vi "75_Vision_RC Servo_DC_Moto_3.vi"() -> ()   [LabVIEW 2018]
uses:
  <userlib>/KNR OS 4.0 LabVIEW Toolkit/Type Definition/Resource.ctl
  <userlib>/KNR OS 4.0 LabVIEW Toolkit/Type Definition/RC Servo Port.ctl
  <userlib>/KNR OS 4.0 LabVIEW Toolkit/Type Definition/DC Motor Port.ctl
panel:
  out "area":dbl
  out "RC Pulse Width (uS)":u16[](array[numeric])
  out "Image Out":T1(plugin-control)
  in  "stop":bool
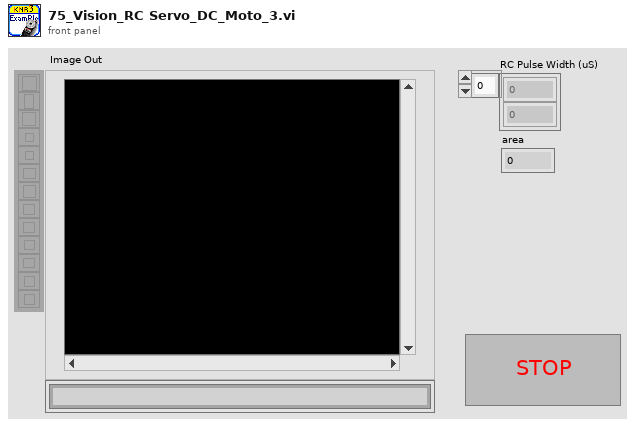
[diagram p1: front panel]
types:
  T1 = typedef "IMAQ Image.ctl" = refnum<image>
  T2 = typedef "DC Motor Port.ctl" = u16
  T3 = typedef "RC Servo Port.ctl" = u16
  T4 = typedef "Resource.ctl" = enum16{"KNRm_DDRC", "KNRm_DDDD", "KNRm_DDDR", "KNRm_DDDC", "KNR", "KNRm_neww"}
  T5 = typedef "KNR3 Reference.ctl" = cluster{"FPGA Session":refnum<class "FPGA Interface Base.lvclass">, "Resource":T4}
  T6 = cluster{"Left":dbl, "Top":dbl, "Right":dbl, "Bottom":dbl}
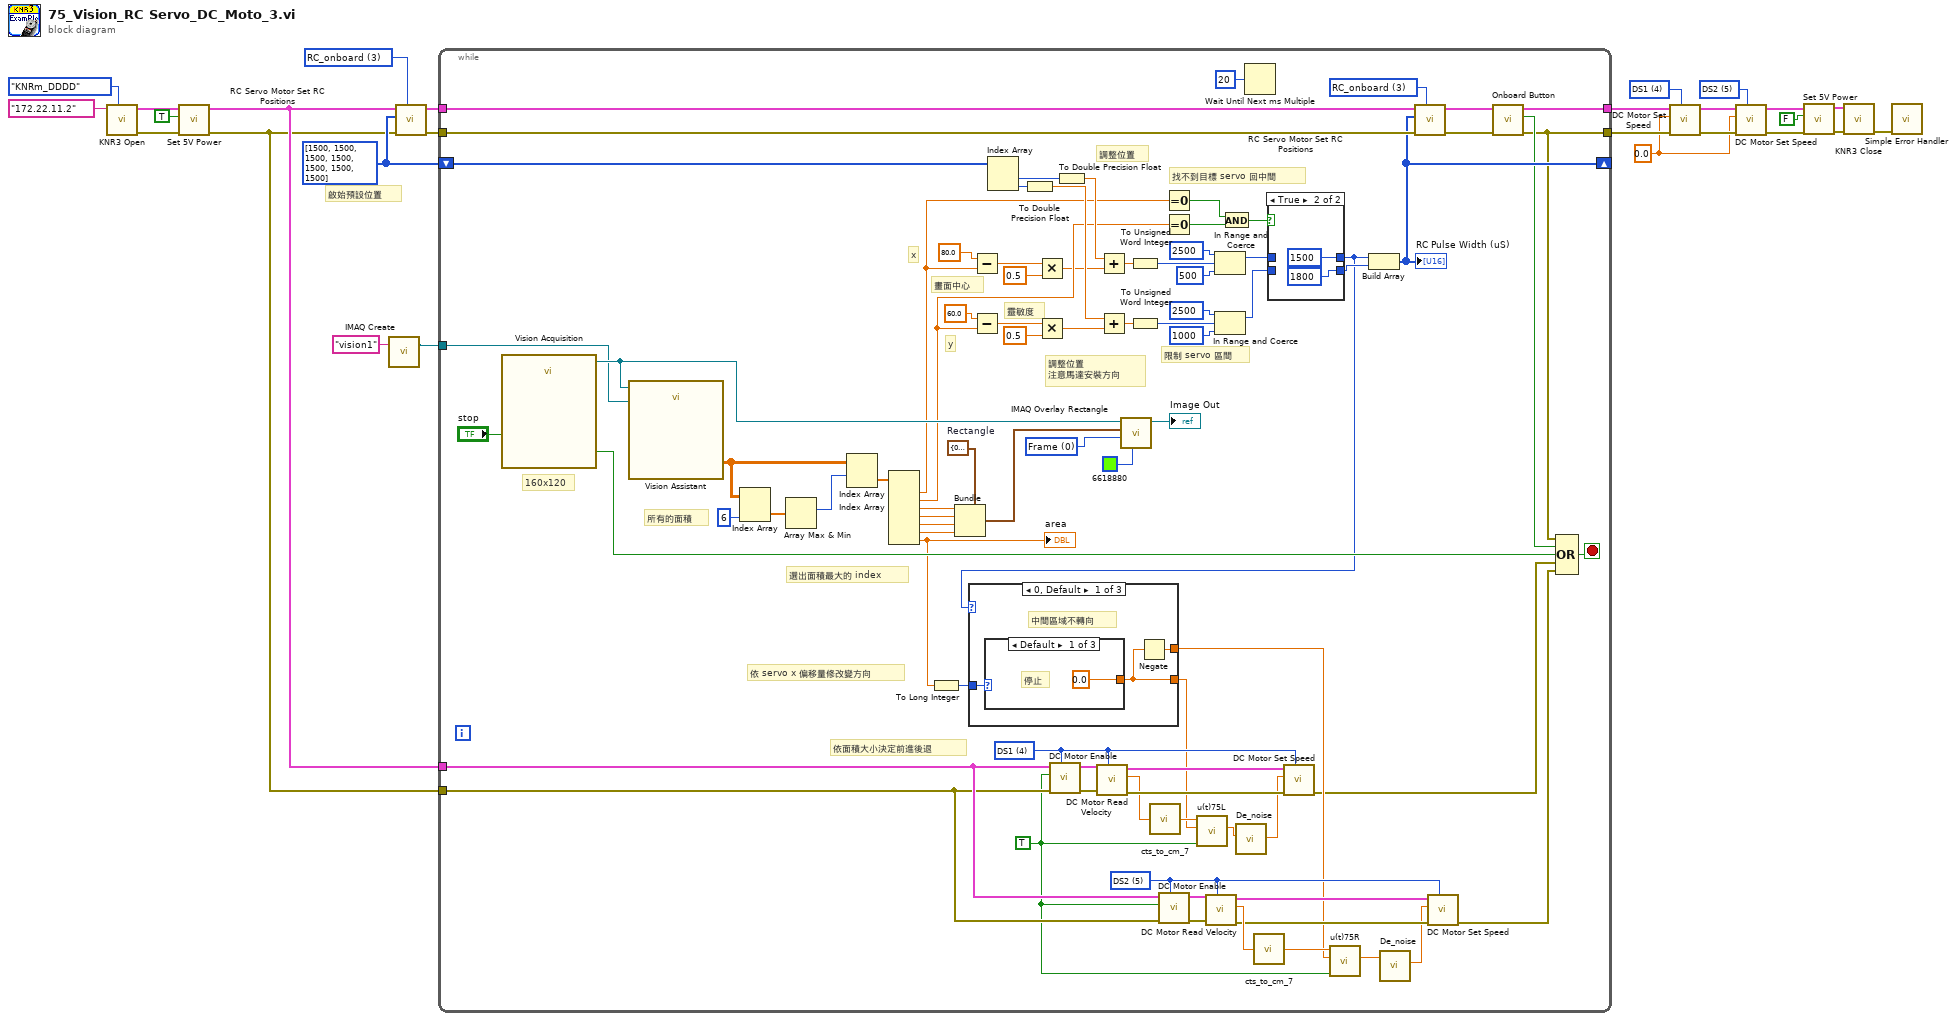
[diagram p0: block diagram]
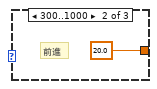
[diagram p2: hidden frame]
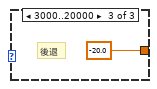
[diagram p3: hidden frame]
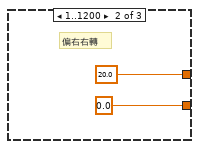
[diagram p4: hidden frame]
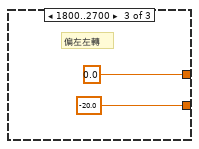
[diagram p5: hidden frame]
diagram:
  w1 = T2 5 items=["DS1"=4, "DS2"=5, "DS3"=6, "DS4"=7] ("Port (DS1)")
  w2 = T2 4 items=["DS1"=4, "DS2"=5, "DS3"=6, "DS4"=7] ("Port (DS1)")
  w3 = 0.0 ("Speed (+-100%)")
  w13 = u16[] [1500, 1500, 1500, 1500, 1500, 1500, 1500] ("RC Pulse Width (1500 uS)")
  w16 = T3 3 items=["RC_onboard"=3, "RC_box"=9] ("Port (RC_onboard)")
  # "啟始預設位置"
  n1 = call <userlib>:"KNR3 Open.vi"("Resource"=Resource."KNRm_DDDD", "IP"="172.22.11.2") -> ("error out"=w22:errorcluster, "KNR out"=w23:T5)  [unwired: 8 in]
  n2 = call <userlib>:"Set 5V Power.vi"("error in (no error)"=w22, "5V Power(T)"=TRUE ("5V Power"), "KNR in"=w23) -> ("error out"=w11:errorcluster, "KNR out"=w12:T5)  [unwired: 7 in]
  n3 = call "IMAQ Create"("Image Name"="vision1") -> ("New Image"=w14:T1)  [unwired: 4 in, 1 out]
  n4 = call <userlib>:"RC Servo Motor Set RC Positions.vi"("Port (RC_onboard)"=w16, "RC Pulse Width (1500 uS)"=w13, "KNR in"=w12) -> ("KNR out"=w17:T5)  [unwired: 7 in, 1 out]
  n5 = while {
    tunnel: w17 -> [w108]
    tunnel: [w35] -> w10
    tunnel: w11 -> [w106]
    tunnel: [w33] -> w9
    tunnel: w14 -> [w88]
    shift-right: [w72] -> _
    shift-left: w13 -> [w75]
    tunnel: w12 -> [w40]
    tunnel: w11 -> [w39]
    stop <- w105 stop-if-true
    w38 = u32 0 items=["Frame", "Fill", "Highlight"] ("Drawing Mode (Frame)")
    w42 = T2 5 items=["DS1"=4, "DS2"=5, "DS3"=6, "DS4"=7] ("Port 2")
    w36 = TRUE ("Enable Motor(F)")
    w55 = T2 4 items=["DS1"=4, "DS2"=5, "DS3"=6, "DS4"=7] ("Port 2")
    w101 = T6 {"Left"=0.0, "Top"=0.0, "Right"=0.0, "Bottom"=0.0}  # Rectangle
    w103 = T3 3 items=["RC_onboard"=3, "RC_box"=9] ("RC Motor")
    # "依 servo x 偏移量修改變方向"
    # "依面積大小決定前進後退"
    # "調整位置\n注意馬達安裝方向"
    # "調整位置"
    # "靈敏度"
    # "所有的面積"
    # "畫面中心"
    # "限制 servo 區間"
    # "找不到目標 servo 回中間"
    # "y"
    # "x"
    # "160x120"
    # "選出面積最大的 index"
    n6 = call "Vision Acquisition"("Stop (F)"="stop") -> ("Image Out"=w93:T1, "Stopped"=w86:bool)  [unwired: 24 in, 1 out]
    n7 = call "Vision Assistant"("Image In"=w93, "Image Dst"=w88) -> ("Particle Measurements (Pixels) (Particle Analysis 1)"=w92:dbl[][])  [unwired: 22 in, 3 out]
    n8 = Index Array "Index Array"(array=w92, index (col)=6 ("disabled index (col)")) -> (element=w91:dbl[])  [unwired: 1 in]
    n9 = Array Max & Min(array=w91) -> (max index (indices)=w90:i32)  [unwired: 3 out]
    n10 = Index Array "Index Array"(array=w92, index (row)=w90) -> (element=w102:dbl[])  [unwired: 1 in]
    n11 = Index Array "Index Array"(array=w102) -> (element #1=w65:dbl, element #2=w64:dbl, element #3=w100:dbl, element #4=w99:dbl, element #5=w98:dbl, element #6=w97:dbl, element #7=w49:dbl)  [unwired: 7 in]
    "area" <- w49
    n12 = To Long Integer(number=w49) -> (32bit integer=w27:i32)
    n13 = Bundle "Bundle"(cluster=w101, "Left"=w100, "Top"=w99, "Right"=w98, "Bottom"=w97) -> (w96:T6)
    n14 = Subtract(x=80.0 ("y"), y=w65) -> (x-y=w82:dbl)
    n15 = Subtract(x=60.0 ("y"), y=w64) -> (x-y=w83:dbl)
    n16 = Index Array "Index Array"(array=w75) -> (element #1=w74:u16, element #2=w73:u16)  [unwired: 2 in]
    n17 = To Double Precision Float(number=w73) -> (double precision float=w66:dbl)
    n18 = Multiply(x=w82, y=0.5) -> (x*y=w63:dbl)
    n19 = Multiply(x=w83, y=0.5) -> (x*y=w62:dbl)
    n20 = call <userlib>:"DC Motor Enable.vi"("Port (DS1)"=w55, "error in (no error)"=w39, "Enable Motor(F)"=w36, "KNR in"=w40) -> ("error out"=w51:errorcluster, "KNR out"=w50:T5)  [unwired: 6 in]
    n21 = To Double Precision Float(number=w74) -> (double precision float=w67:dbl)
    n22 = call <userlib>:"DC Motor Read Velocity.vi"("Port (DS1)"=w55, "error in (no error)"=w51, "KNR in"=w50) -> ("error out"=w54:errorcluster, "Velocity (cts/sec)"=w52:dbl, "KNR out"=w53:T5)  [unwired: 6 in]
    n23 = Add(x=w67, y=w63) -> (x+y=w84:dbl)
    n24 = Add(x=w66, y=w62) -> (x+y=w85:dbl)
    n25 = call "IMAQ Overlay Rectangle"("Color"=u32 6618880, "Drawing Mode (Frame)"=w38, "Rectangle"=w96, "Image"=w93) -> ("Image Out"=→"Image Out":T1)  [unwired: 6 in, 1 out]
    n26 = To Unsigned Word Integer(number=w84) -> (unsigned 16bit integer=w69:u16)
    n27 = To Unsigned Word Integer(number=w85) -> (unsigned 16bit integer=w68:u16)
    n28 = call "cts_to_cm_7.vi"("cts"=w52) -> ("cm"=w37:dbl)
    n29 = call <userlib>:"DC Motor Enable.vi"("Port (DS1)"=w42, "error in (no error)"=w39, "Enable Motor(F)"=w36, "KNR in"=w40) -> ("error out"=w46:errorcluster, "KNR out"=w47:T5)  [unwired: 6 in]
    n30 = Equal To 0?(x=w65) -> (x = 0?=w59:bool)
    n31 = Equal To 0?(x=w64) -> (x = 0?=w60:bool)
    n32 = call <userlib>:"DC Motor Read Velocity.vi"("Port (DS1)"=w42, "error in (no error)"=w46, "KNR in"=w47) -> ("error out"=w43:errorcluster, "Velocity (cts/sec)"=w45:dbl, "KNR out"=w44:T5)  [unwired: 6 in]
    n33 = In Range and Coerce(upper limit=u16 2500, x=w69, lower limit=u16 500) -> (coerced(x)=w58:u16)  [unwired: 1 out]
    n34 = In Range and Coerce(upper limit=u16 2500, x=w68, lower limit=u16 1000) -> (coerced(x)=w57:u16)  [unwired: 1 out]
    n35 = And(x=w59, y=w60) -> (x .and. y?=w61:bool)
    n36 = Wait Until Next ms Multiple(millisecond multiple=u32 20) -> ()  [unwired: 1 out]
    n37 = call "cts_to_cm_7.vi"("cts"=w45) -> ("cm"=w48:dbl)
    n38 = case shown="True" w61 {
      tunnel: w58 -> [w120 _]
      tunnel: w57 -> [w119 _]
      tunnel: [w120 u16 1500] -> w28
      tunnel: [w119 u16 1800] -> w56
      frame False {
      }
      frame True {
      }
    }
    n39 = case shown="0, Default" w28 {
      tunnel: [w110 0.0 -20.0] -> w26
      tunnel: [w111 20.0 0.0] -> w25
      tunnel: w27 -> [w109 _ _]
      frame 0, Default {
        # "中間區域不轉向"
        n40 = case shown="Default" w109 {
          tunnel: [0.0 20.0 -20.0] -> w110
          frame Default {
            # "停止"
          }
          frame 300..1000 {
            # "前進"
          }
          frame 3000..20000 {
            # "後退"
          }
        }
        n41 = Negate(x=w110) -> (-x=w111:dbl)
      }
      frame 1..1200 {
        # "偏右右轉"
      }
      frame 1800..2700 {
        # "偏左左轉"
      }
    }
    n42 = call "u(t)75L.vi"("Velocity"=w37, "Desire Velosity"=w26, "enable"=w36) -> ("u(t)"=w31:dbl)  [unwired: 7 in]
    n43 = call "De_noise.vi"("u(t)"=w31) -> ("u(t)2"=w32:dbl)  [unwired: 6 in]
    n44 = call <userlib>:"DC Motor Set Speed.vi"("Port (DS1)"=w55, "error in (no error)"=w54, "Speed (+-100%)"=w32, "KNR in"=w53) -> ("error out"=w24:errorcluster)  [unwired: 6 in, 1 out]
    n45 = call "u(t)75R.vi"("Velocity"=w48, "Desire Velosity"=w25, "enable"=w36) -> ("u(t)"=w30:dbl)  [unwired: 7 in]
    n46 = Build Array "Build Array"(w28, w56) -> (w72:u16[])
    "RC Pulse Width (uS)" <- w72
    n47 = call "De_noise.vi"("u(t)"=w30) -> ("u(t)2"=w29:dbl)  [unwired: 6 in]
    n48 = call <userlib>:"RC Servo Motor Set RC Positions.vi"("Port (RC_onboard)"=w103, "error in (no error)"=w106, "RC Pulse Width (1500 uS)"=w72, "KNR in"=w108) -> ("error out"=w33:errorcluster, "KNR out"=w107:T5)  [unwired: 6 in]
    n49 = call <userlib>:"DC Motor Set Speed.vi"("Port (DS1)"=w42, "error in (no error)"=w43, "Speed (+-100%)"=w29, "KNR in"=w44) -> ("error out"=w41:errorcluster)  [unwired: 6 in, 1 out]
    n50 = call <userlib>:"Onboard Button.vi"("KNR in"=w107) -> ("value"=w34:bool, "KNR out"=w35:T5)  [unwired: 8 in, 1 out]
    n51 = Compound Arithmetic op=OR(w33, w34, w86, w24, w41) -> (w105:bool)
  }
  n52 = call <userlib>:"DC Motor Set Speed.vi"("Port (DS1)"=w2, "Speed (+-100%)"=w3, "KNR in"=w10) -> ("KNR out"=w5:T5)  [unwired: 7 in, 1 out]
  n53 = call <userlib>:"DC Motor Set Speed.vi"("Port (DS1)"=w1, "Speed (+-100%)"=w3, "KNR in"=w5) -> ("KNR out"=w4:T5)  [unwired: 7 in, 1 out]
  n54 = call <userlib>:"Set 5V Power.vi"("error in (no error)"=w9, "5V Power(T)"=FALSE, "KNR in"=w4) -> ("error out"=w7:errorcluster, "KNR out"=w8:T5)  [unwired: 7 in]
  n55 = call <userlib>:"KNR3 Close.vi"("error in (no error)"=w7, "KNR in"=w8) -> ("error out"=w21:errorcluster)  [unwired: 9 in]
  n56 = call <vilib>:"Simple Error Handler.vi"("error in (no error)"=w21) -> ()  [unwired: 4 in, 5 out]
